vi "Run Output Actor Hardware.vi"(8 "error in (no error)":errorcluster, 11 "Output Actor Hardware":refnum<class "Output Actor Hardware.lvclass">) -> (0 "error out":errorcluster, 3 "Output Actor Hardware Interface":refnum<class "Output Actor Hardware Interface.lvclass">)   [LabVIEW 2015, in "Output Actor Hardware.lvclass"]
uses:
  Output Actor Hardware.lvclass
  Output Actor Hardware Interface/Output Actor Hardware Interface.lvclass
  Output Actor/Output Actor Interface/Output Actor Interface.lvclass
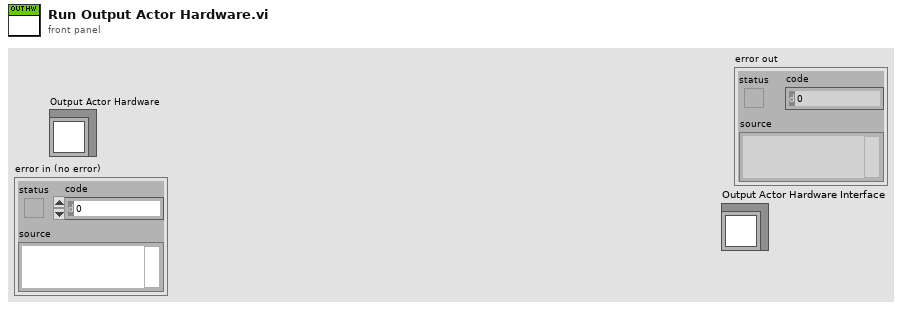
[diagram p1: front panel]
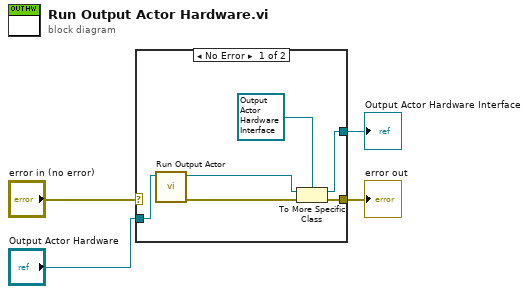
[diagram p0: block diagram]
diagram:
  n1 = case shown="No Error" "error in (no error)" {
    selector: "error in (no error)" -> [_ w11]
    tunnel: "Output Actor Hardware" -> [w10 _]
    tunnel: [w6 w11] -> w3
    tunnel: [w5 _] -> w1
    frame No Error {
      n2 = call "Run Output Actor.vi"("output_actor.lvclass"=w10) -> ("error out"=w9:errorcluster, "Output Actor Interface"=w8:refnum<class "Output Actor Interface.lvclass">)  [unwired: 9 in]
      n3 = To More Specific Class(target class=refnum<class "Output Actor Hardware Interface.lvclass"> refnum ("Output Actor Hardware Interface.lvclass"), reference=w8, error in=w9) -> (specific class reference=w5:refnum<class "Output Actor Hardware Interface.lvclass">, error out=w6:errorcluster)
    }
    frame Error {
    }
  }
  "error out" <- w3
  "Output Actor Hardware Interface" <- w1
